vi "openQCM with film resistance .vi"() -> ()   [LabVIEW 2014]
uses:
  <vilib>/Analysis/baseanly.llb/Mean (DBL).vi
  <vilib>/Instr/_visa.llb/VISA Configure Serial Port (Instr).vi
  <vilib>/Utility/file.llb/Write To Spreadsheet File (string).vi
  <vilib>/Analysis/NI_AALBase.lvlib
panel:
  out "resistance chart":dbl(graph)
  in  "Arduino address":refnum<visa-resource-name>
  out "Measurements":T1 {"Frequency (Hz)" format="%#_12g"}
  in  "Save data?":bool
  out "frequency chart":dbl(graph)
  in  "Cluster":T2
  in  "Stop Button":bool
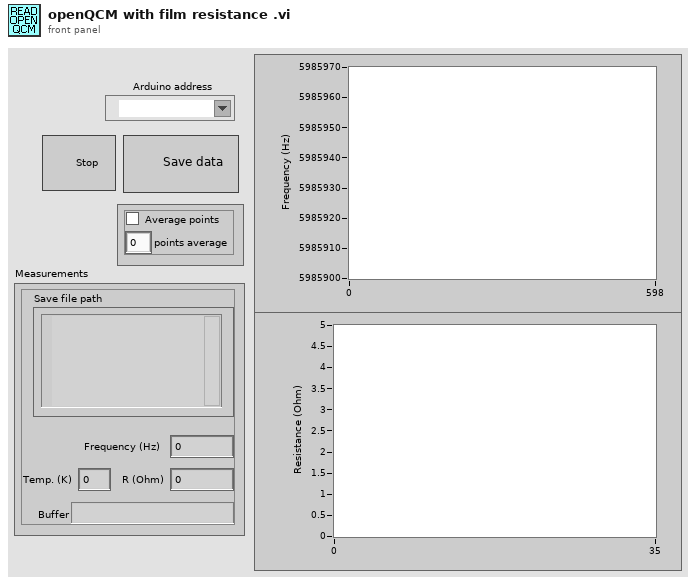
[diagram p1: front panel]
types:
  T1 = cluster{"Frequency (Hz)":dbl, "Temp. (K)":dbl, "Buffer":string, "R (Ohm)":dbl, "Save file path":path}
  T2 = cluster{"points average":i32, "average points?":bool}
  T3 = enum16{"open", "replace", "create", "open or create", "replace or create", "replace or create with confirmation"}
  T4 = cluster{dbl, dbl, "read buffer":string, dbl, path}
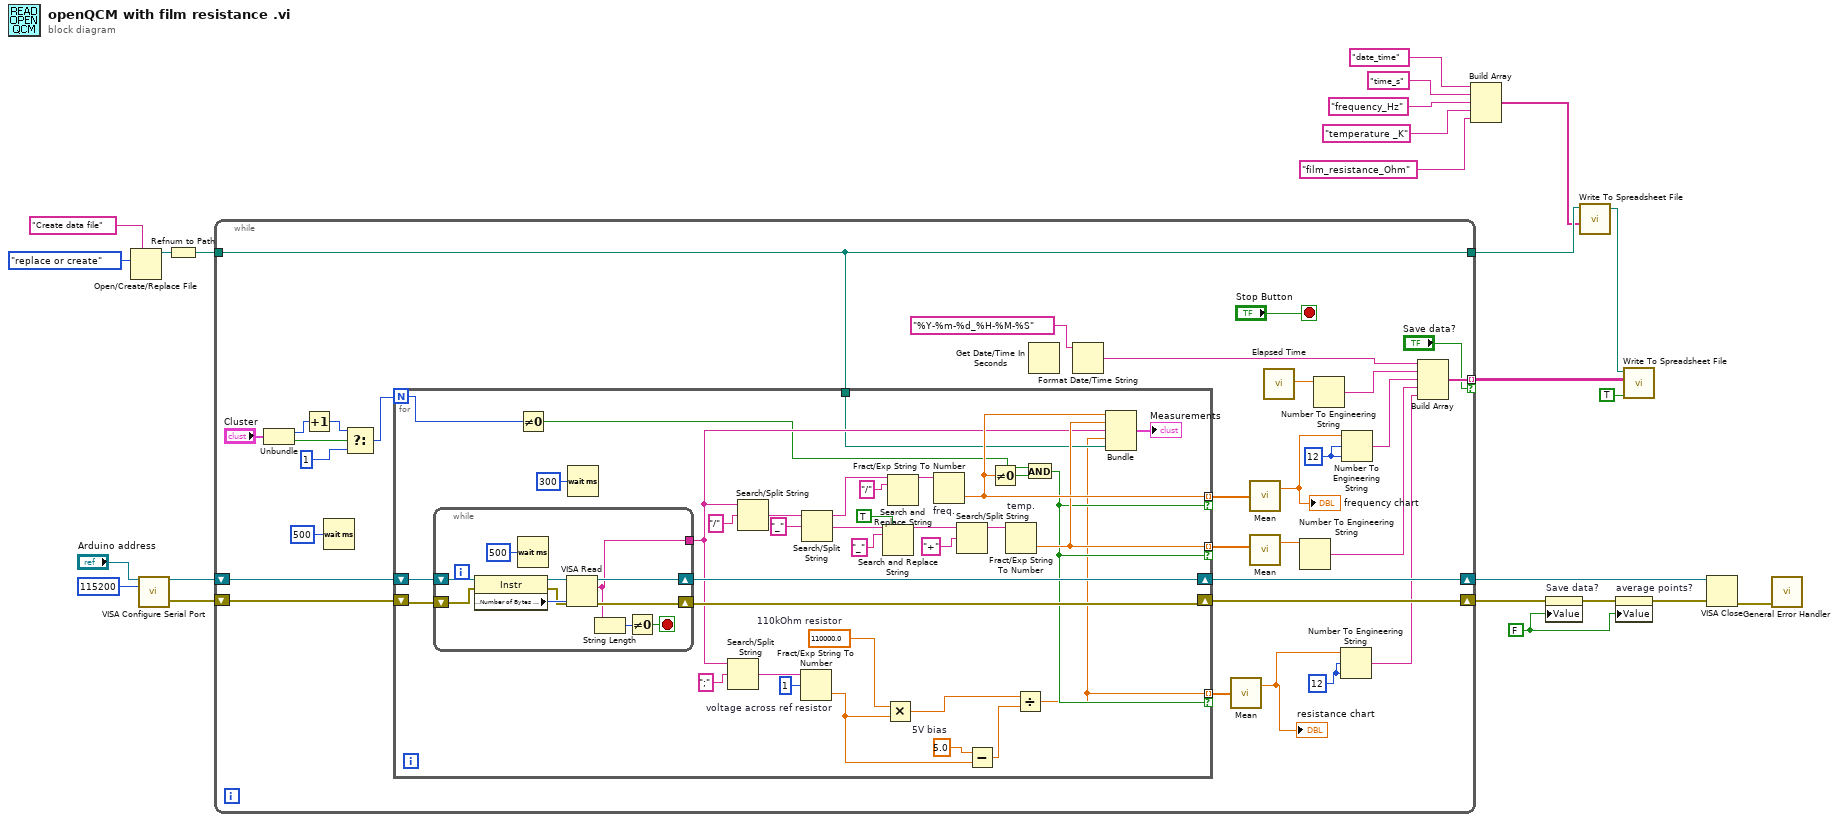
[diagram p0: block diagram]
diagram:
  w6 = FALSE ("Save data?")
  n1 = Open/Create/Replace File(prompt="Create data file", operation (0:open)=T3."replace or create") -> (refnum out=w14:refnum<file>)  [unwired: 4 in, 2 out]
  n2 = call-poly "VISA Configure Serial Port"("VISA resource name"="Arduino address", "baud rate (9600)"=u32 115200) -> ("VISA resource name out"=w22:refnum<visa-resource-name>, "error out"=w21:errorcluster)  [unwired: 12 in]
  n3 = Refnum to Path(1:w14) -> (0:w4:path)
  n4 = while {
    shift-right: [w54] -> w23
    shift-left: w22 -> [w52]
    shift-right: [w53] -> w8
    shift-left: w21 -> [w51]
    tunnel: [w38] -> w20 mode=indexing if="Save data?"
    tunnel: [w28] -> w17
    tunnel: w4 -> [w28]
    stop <- "Stop Button" stop-if-true
    w25 = 12 ("offset")
    w46 = 12 ("offset")
    n5 = Unbundle("Cluster") -> ("points average"=w33:i32, "average points?"=w30:bool)
    n6 = Increment(x=w33) -> (x+1=w31:i32)
    n7 = Wait (ms)(milliseconds to wait=u32 500) -> ()  [unwired: 1 out]
    n8 = Select(t=w31, s=w30, f=1) -> (s? t:f=w40:i32)
    n9 = for {
      N: w40 -> [w64]
      tunnel: [w75] -> w48 mode=indexing if=w61
      shift-right: [w73] -> w54
      shift-left: w52 -> [w78]
      shift-right: [w72] -> w53
      shift-left: w51 -> [w77]
      tunnel: [w74] -> w36 mode=indexing if=w61
      tunnel: [w60] -> w29 mode=indexing if=w61
      tunnel: w28 -> [w66]
      w55 = 5.0  # 5V bias
      w56 = 110000.0  # 110kOhm resistor
      n10 = while {
        shift-right: [w96] -> w73
        shift-left: w78 -> [w100]
        shift-right: [w91] -> w72
        shift-left: w77 -> [w99]
        tunnel: [w90] -> w69
        stop <- w94 stop-if-true
        # "wait until bytes are ready"
        n11 = property class="Instr"(reference=w100, error in=w99) -> (reference out=w97:refnum<visa-resource-name>, error out=w92:errorcluster, "Serial Settings:Number of Bytes at Serial Port"=w95:u32)
        n12 = Wait (ms)(milliseconds to wait=u32 500) -> ()  [unwired: 1 out]
        n13 = VISA Read(VISA resource name=w97, byte count=w95, error in (no error)=w92) -> (VISA resource name out=w96:refnum<visa-resource-name>, read buffer=w90:string, error out=w91:errorcluster)  [unwired: 1 out]
        n14 = String Length(string=w90) -> (length=w93:i32)
        n15 = Not Equal To 0?(x=w93) -> (x != 0?=w94:bool)
      }
      n16 = Not Equal To 0?(x=w64) -> (x != 0?=w62:bool)
      n17 = Wait (ms)(milliseconds to wait=u32 300) -> ()  [unwired: 1 out]
      n18 = Search/Split String(string=w69, search string/char (-)=";") -> (match + rest of string=w68:string)  [unwired: 1 in, 2 out]
      n19 = Search/Split String(string=w69, search string/char (-)="/") -> (match + rest of string=w84:string)  [unwired: 1 in, 2 out]
      n20 = Fract/Exp String To Number "voltage across ref resistor"(string=w68, offset=1) -> (number=w57:dbl)  [unwired: 2 in, 1 out]
      n21 = Search/Split String(string=w84, search string/char (-)="_") -> (substring before match=w89:string, match + rest of string=w85:string)  [unwired: 1 in, 1 out]
      n22 = Search and Replace String(replace all?=TRUE ("replace all? (F)"), input string=w85, search string="_") -> (result string=w79:string)  [unwired: 5 in, 3 out]
      n23 = Multiply(x=w56, y=w57) -> (x*y=w59:dbl)
      n24 = Search and Replace String(input string=w89, search string="/" ("replace string (\"\")")) -> (result string=w81:string)  [unwired: 6 in, 3 out]
      n25 = Fract/Exp String To Number "freq."(string=w81) -> (number=w75:dbl)  [unwired: 3 in, 1 out]
      n26 = Search/Split String(string=w79, search string/char (-)="+") -> (substring before match=w71:string)  [unwired: 1 in, 2 out]
      n27 = Subtract(x=w55, y=w57) -> (x-y=w58:dbl)
      n28 = Not Equal To 0?(x=w75) -> (x != 0?=w63:bool)
      n29 = Fract/Exp String To Number "temp."(string=w71) -> (number=w74:dbl)  [unwired: 3 in, 1 out]
      n30 = Divide(x=w59, y=w58) -> (x/y=w60:dbl)
      n31 = And(x=w62, y=w63) -> (x .and. y?=w61:bool)
      n32 = Bundle(w75, w74, "read buffer"=w69, w60, w66) -> (→"Measurements":T4)  [unwired: 1 in]
    }
    n33 = Get Date/Time In Seconds() -> ()  [unwired: 1 out]
    n34 = Format Date/Time String(time format string (%c)="%Y-%m-%d_%H-%M-%S") -> (date/time string=w44:string)  [unwired: 2 in]
    n35 = call-poly <vilib>:"Mean.vi"("X"=w29) -> ("mean"=w26:dbl)  [unwired: 1 out]
    "resistance chart" <- w26
    n36 = call-poly <vilib>:"Mean.vi"("X"=w48) -> ("mean"=w42:dbl)  [unwired: 1 out]
    "frequency chart" <- w42
    n37 = call-poly <vilib>:"Mean.vi"("X"=w36) -> ("mean"=w35:dbl)  [unwired: 1 out]
    n38 = call "Elapsed Time"() -> ("Elapsed Time (s)"=w45:dbl)  [unwired: 12 in, 7 out]
    n39 = Number To Engineering String(4:w35) -> (0:w34:string)  [unwired: 3 in]
    n40 = Number To Engineering String(4:w45) -> (0:w43:string)  [unwired: 3 in]
    n41 = Number To Engineering String(2:w25, 3:w25, 4:w26) -> (0:w27:string)  [unwired: 1 in]
    n42 = Number To Engineering String(2:w46, 3:w46, 4:w42) -> (0:w41:string)  [unwired: 1 in]
    n43 = Build Array(w44, w43, w41, w34, w27) -> (w38:string[])
  }
  n44 = Build Array("date_time" ("time format string (%c)"), "time_s" ("time format string (%c)"), "frequency_Hz" ("time format string (%c)"), "temperature _K" ("time format string (%c)"), "film_resistance_Ohm" ("time format string (%c)")) -> (w16:string[])
  n45 = property on="Save data?" class="Bool (strict)"(error in=w8, "Value"=w6) -> (error out=w9:errorcluster)  [unwired: 1 in, 1 out]
  n46 = call-poly <vilib>:"Write To Spreadsheet File.vi"("1D data"=w16, "file path (dialog if empty)"=w17) -> ("new file path (Not A Path if cancelled)"=w19:path)  [unwired: 6 in]
  n47 = property on="average points?" class="Bool (strict)"(error in=w9, "Value"=w6) -> (error out=w7:errorcluster)  [unwired: 1 in, 1 out]
  n48 = call-poly <vilib>:"Write To Spreadsheet File.vi"("append to file? (new file:F)"=TRUE, "2D data"=w20, "file path (dialog if empty)"=w19) -> ()  [unwired: 5 in, 1 out]
  n49 = VISA Close(VISA resource name=w23, error in (no error)=w7) -> (error out=w5:errorcluster)
  n50 = call <vilib>:"General Error Handler.vi"("error in (no error)"=w5) -> ()  [unwired: 10 in, 5 out]
